vi "PID_Controller.vi"(0 "Controller Type":string(combo)="PD", 1 "Kp":dbl=57.53, 2 "Kd":dbl=0.07, 3 "Ki":dbl=0.07, 4 "Setpoint":dbl, 5 "Feedback Signal":dbl, 6 "e(t-1).dt":dbl, 7 "t":dbl, 8 "e(t-1)":dbl) -> (14 "Control Signal":dbl, 15 "e(t)":dbl, 16 "e(t-1).dt+e(t).dt":dbl)   [LabVIEW 2021]
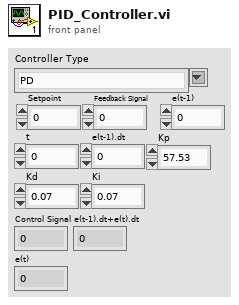
[diagram p1: front panel]
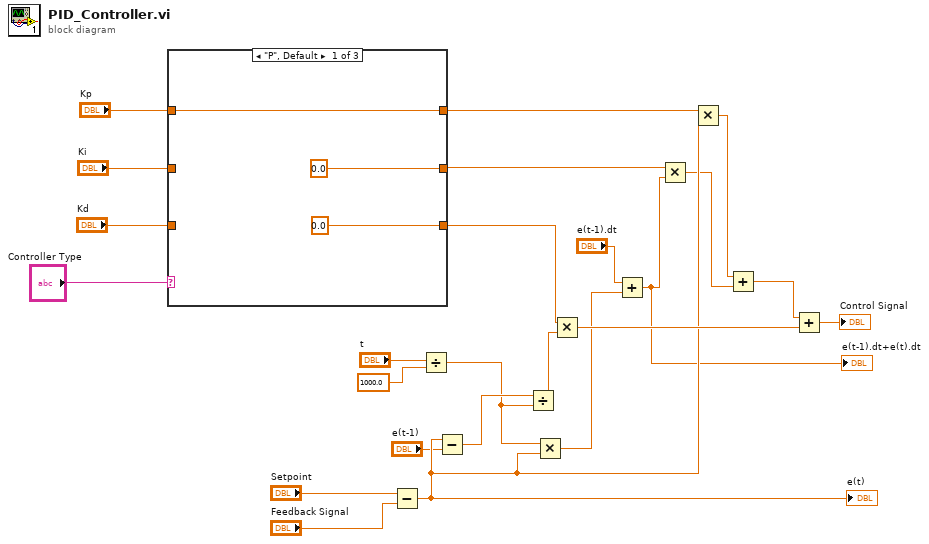
[diagram p0: block diagram]
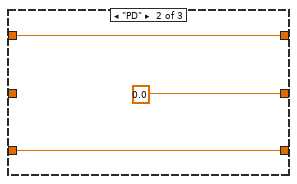
[diagram p2: hidden frame]
diagram:
  n1 = case shown="\"P\", Default" "Controller Type" {
    tunnel: [w26 w29 w33] -> w21
    tunnel: [0.0 ("element") w28 w31] -> w18
    tunnel: [0.0 ("Ti") 0.0 w32] -> w11
    tunnel: "Kp" -> [w26 w29 w33]
    tunnel: "Ki" -> [_ _ w32]
    tunnel: "Kd" -> [_ w28 w31]
    frame "P", Default {
    }
    frame "PD" {
    }
    frame "PID" {
    }
  }
  n2 = Subtract(x="Setpoint", y="Feedback Signal") -> (x-y=w13:dbl)
  "e(t)" <- w13
  n3 = Divide(x="t", y=1000.0) -> (x/y=w7:dbl)
  n4 = Subtract(x=w13, y="e(t-1)") -> (x-y=w17:dbl)
  n5 = Divide(x=w17, y=w7) -> (x/y=w16:dbl)
  n6 = Multiply(x=w7, y=w13) -> (x*y=w4:dbl)
  n7 = Multiply(x=w18, y=w16) -> (x*y=w15:dbl)
  n8 = Add(x="e(t-1).dt", y=w4) -> (x+y=w1:dbl)
  "e(t-1).dt+e(t).dt" <- w1
  n9 = Multiply(x=w11, y=w1) -> (x*y=w2:dbl)
  n10 = Multiply(x=w21, y=w13) -> (x*y=w20:dbl)
  n11 = Add(x=w20, y=w2) -> (x+y=w19:dbl)
  n12 = Add(x=w19, y=w15) -> (x+y=→"Control Signal":dbl)
